vi "set_settings_cluster.vi"(8 "error in (no error)":errorcluster, 10 "settings cluster variant":variant, 11 "TrajectoryDL121017Hopping in":refnum<class "TrajectoryDL121017Hopping.lvclass">) -> (0 "error out":errorcluster, 3 "TrajectoryDL121017Hopping out":refnum<class "TrajectoryDL121017Hopping.lvclass">)   [LabVIEW 2010, in "TrajectoryDL121017Hopping.lvclass"]
uses:
  TrajectoryDL121017Hopping.lvclass
  TrajectoryDL121017Hopping.lvclass/TrajectoryDL121017Hopping.ctl
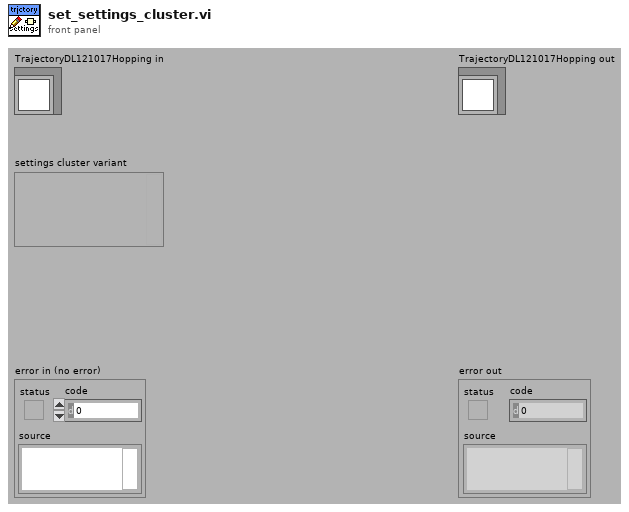
[diagram p1: front panel]
types:
  T1 = typedef "TrajectoryDL121017Hopping.lvclass/settings_cluster.ctl" = cluster{"uncaging time":dbl[unit], "hopping time":dbl[unit], "subpattern type":T2, "spiral parameters":T3}
  T2 = typedef "TrajectoryDL121017Hopping.lvclass/subpattern_type_enum.ctl" = enum16{"none", "spiral"}
  T3 = typedef "TrajectoryDL121017Hopping.lvclass/spiral_parameters_cluster.ctl" = cluster{"diameter":dbl[unit], "number of windings":i32}
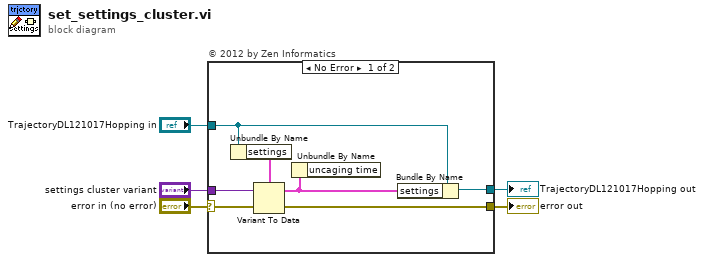
[diagram p0: block diagram]
diagram:
  n1 = case "© 2012 by Zen Informatics" shown="No Error" "error in (no error)" {
    selector: "error in (no error)" -> [w12 w14]
    tunnel: "TrajectoryDL121017Hopping in" -> [w7 w13]
    tunnel: [w6 w13] -> w3
    tunnel: [w11 w14] -> w2
    tunnel: "settings cluster variant" -> [w10 _]
    frame No Error {
      n2 = Unbundle By Name(w7) -> ("settings"=w9:T1)
      n3 = Variant To Data(error in=w12, Variant=w10, type=w9) -> (error out=w11:errorcluster, data=w8:T1)
      n4 = Unbundle By Name(w8) -> ()  [unwired: 1 out]
      n5 = Bundle By Name(cluster=w7, "settings"=w8) -> (w6:refnum<class "TrajectoryDL121017Hopping.lvclass">)
    }
    frame Error {
    }
  }
  "error out" <- w2
  "TrajectoryDL121017Hopping out" <- w3
